vi "temp.vi"() -> ()   [LabVIEW 2025]
panel:
  out "output array":string[](array[string])
  out "String":string
  in  "100 Samples":string[](array[string])
  in  "10000 Samples":dbl[](array[numeric])
  out "error out":errorcluster
  in  "decimal integer string 2":string[](array[string])
  out "decimal integer string":string[](array[string])
  in  "file path (use dialog)":path
  out "Output":dbl[](array[numeric])
  out "x-y*floor(x/y)":i32
  out "floor(x/y)":i32
  out "Elapsed_time":dbl format="%<%H:%M:%S%2u>t"
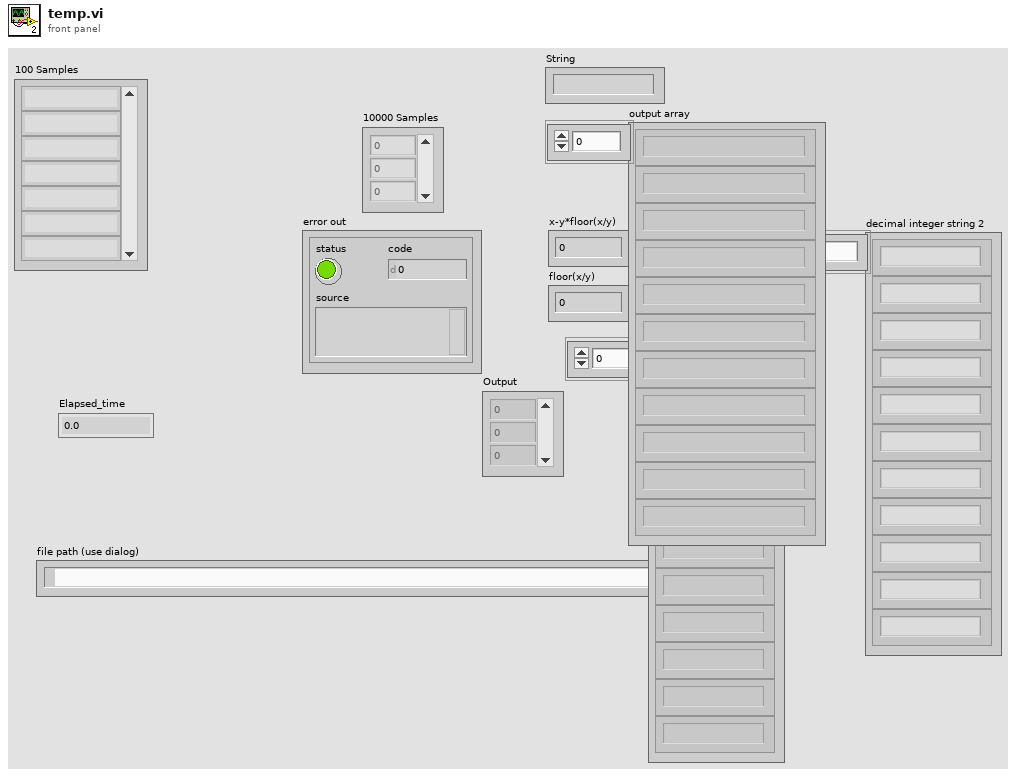
[diagram p1: front panel]
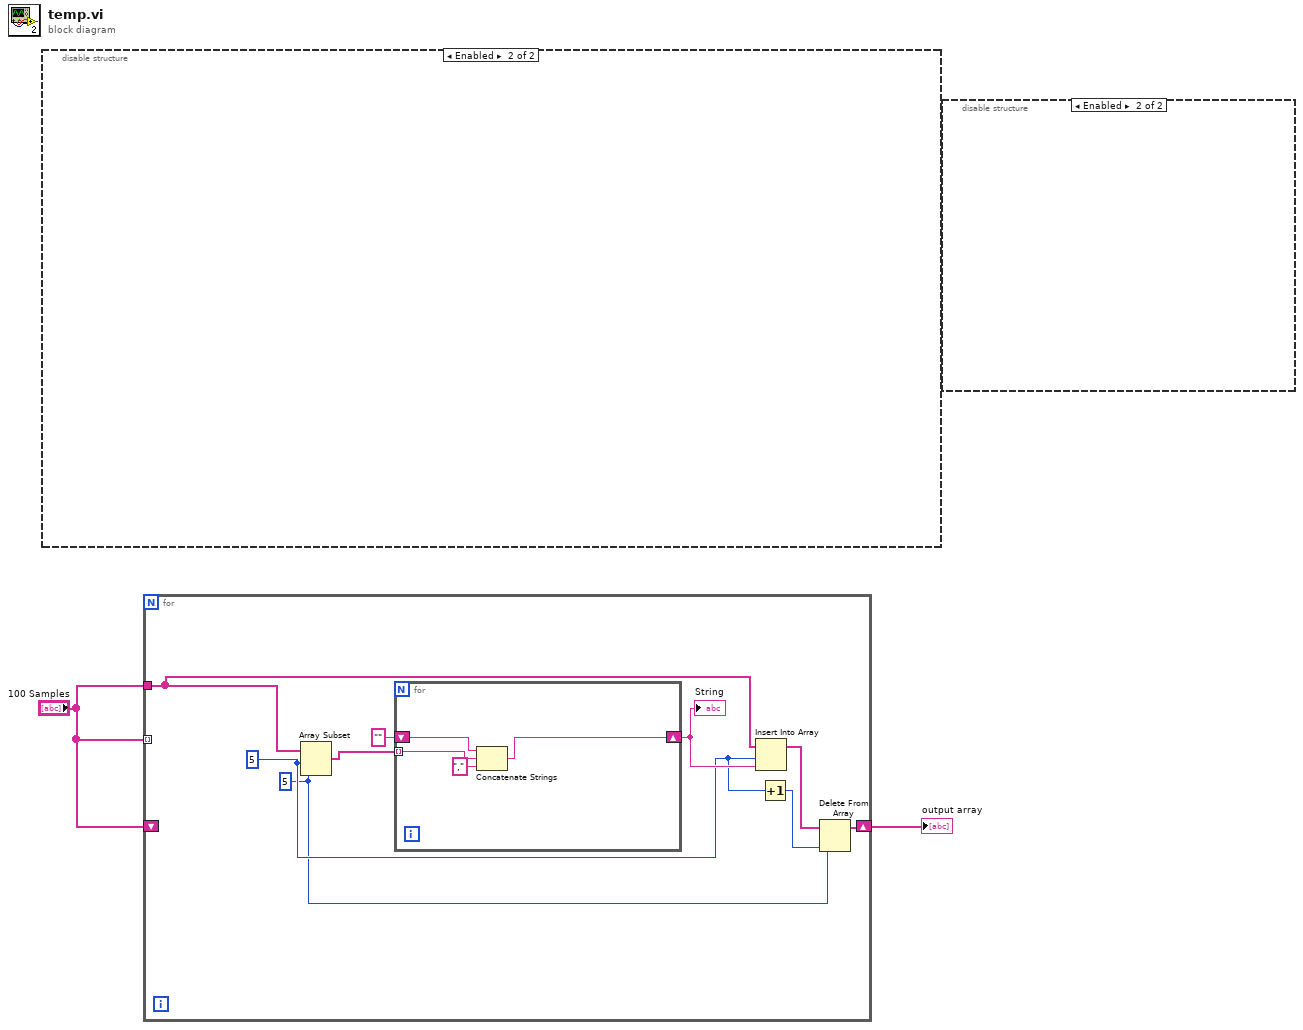
[diagram p0: block diagram]
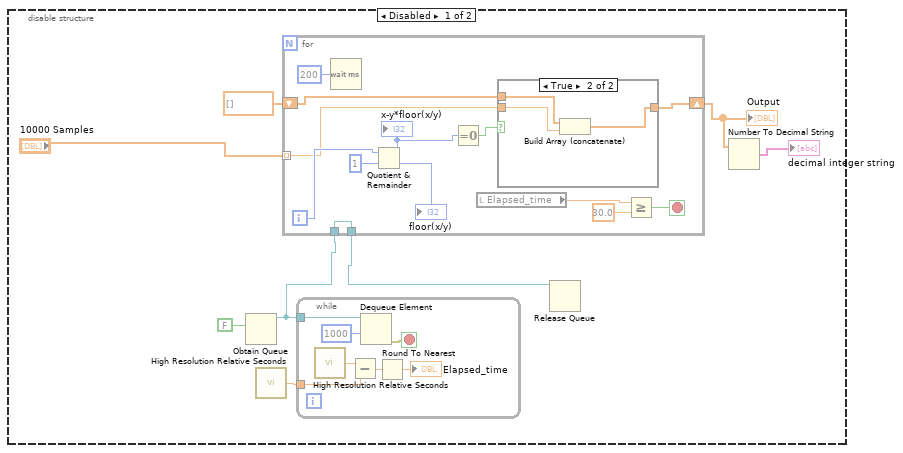
[diagram p2: hidden frame]
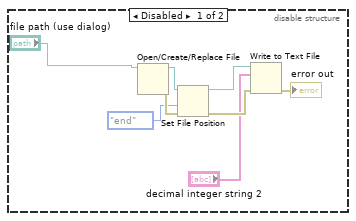
[diagram p4: hidden frame]
diagram:
  n1 = disable-structure shown="Enabled" {
    frame Disabled {
      n2 = Obtain Queue(element data type=FALSE) -> (queue out=w8:refnum<queue>)  [unwired: 4 in, 2 out]
      n3 = call <vilib>:"High Resolution Relative Seconds.vi"() -> ("relative seconds"=w10:dbl)
      n4 = for {
        tunnel: "10000 Samples" -> [w23] mode=indexing
        tunnel: w8 -> [w30]
        tunnel: [w30] -> w7
        shift-right: [w22] -> w5
        shift-left: dbl[] [] -> [w21]
        i -> [w26]
        stop <- w18 stop-if-true
        n5 = Wait (ms)(milliseconds to wait=u32 200) -> ()  [unwired: 1 out]
        n6 = Quotient & Remainder(x=w26, y=1) -> (x-y*floor(x/y)=w25:i32, floor(x/y)=→"floor(x/y)":i32)
        "x-y*floor(x/y)" <- w25
        n7 = Equal To 0?(x=w25) -> (x = 0?=w24:bool)
        n8 = local read "Elapsed_time"() -> (w20:dbl)
        n9 = case shown="True" w24 {
          tunnel: w23 -> [_ w33]
          tunnel: [w31 w34] -> w22
          tunnel: w21 -> [w31 w32]
          frame False {
          }
          frame True {
            n10 = Build Array (concatenate)(w32, w33) -> (w34:dbl[])
          }
        }
        n11 = Greater Or Equal?(x=w20, y=30.0) -> (x >= y?=w18:bool)
      }
      "Output" <- w5
      n12 = while {
        tunnel: w10 -> [w15]
        tunnel: w8 -> [w14]
        stop <- w12 stop-if-true
        n13 = call <vilib>:"High Resolution Relative Seconds.vi"() -> ("relative seconds"=w16:dbl)
        n14 = Subtract(x=w16, y=w15) -> (x-y=w17:dbl)
        n15 = Dequeue Element(queue=w14, timeout in ms (-1)=1000) -> (error out=w12:errorcluster)  [unwired: 1 in, 3 out]
        n16 = Round To Nearest(number=w17) -> (nearest integer value=→"Elapsed_time":dbl)
      }
      n17 = Release Queue(queue=w7) -> ()  [unwired: 2 in, 3 out]
      n18 = Number To Decimal String(number=w5) -> (decimal integer string=→"decimal integer string":string[])  [unwired: 1 in]
    }
    frame Enabled {
    }
  }
  n19 = for {
    tunnel: "100 Samples" -> [_] mode=indexing
    shift-right: [w36] -> w2
    shift-left: "100 Samples" -> [_]
    tunnel: "100 Samples" -> [w35]
    w37 = 5 ("length")
    w39 = 5 ("index")
    n20 = Array Subset(array=w35, index=w39, length=w37) -> (w43:string[])
    n21 = for {
      tunnel: w43 -> [w47] mode=indexing
      shift-right: [w46] -> w41
      shift-left: "" -> [w45]
      n22 = Concatenate Strings(w45, w47, "," ("string")) -> (w46:string)
    }
    "String" <- w41
    n23 = Insert Into Array(array=w35, index=w39, new element=w41) -> (w40:string[])
    n24 = Increment(x=w39) -> (x+1=w38:i32)
    n25 = Delete From Array(array=w40, length=w37, index=w38) -> (array with subset deleted=w36:string[])  [unwired: 1 out]
  }
  "output array" <- w2
  n26 = disable-structure shown="Enabled" {
    frame Disabled {
      n27 = Open/Create/Replace File(file path (use dialog)="file path (use dialog)") -> (refnum out=w50:refnum<file>, error out=w55:errorcluster)  [unwired: 5 in, 1 out]
      n28 = Set File Position(refnum=w50, from (0:start)=enum16{"start", "end", "current"}."end", error in=w55) -> (refnum out=w49:refnum<file>, error out=w53:errorcluster)  [unwired: 1 in]
      n29 = Write to Text File(file (use dialog)=w49, text="decimal integer string 2", error in=w53) -> (error out=→"error out":errorcluster)  [unwired: 1 in, 2 out]
    }
    frame Enabled {
    }
  }
